vi "Multiple_File_Opener_Tester2.vi"() -> ()   [LabVIEW 2023]
uses:
  <vilib>/Utility/file.llb/Read Delimited Spreadsheet (string).vi
  <vilib>/Utility/file.llb/Read Delimited Spreadsheet (DBL).vi
panel:
  out "latest notification":string
  in  "Base Folder 2":path=path "C:/Users/AIIH/Documents/LabVIEW/EEG/Filtered_Data"
  in  "Boolean":bool
  in  "Files":path=path "C:/Users/AIIH/Documents/LabVIEW/EEG/RECORDS_1.csv"
  in  "stop":bool
  out "Header of EEGs":string[](array[string])
  out "Dataset of EEGs":dbl[][](array[numeric])
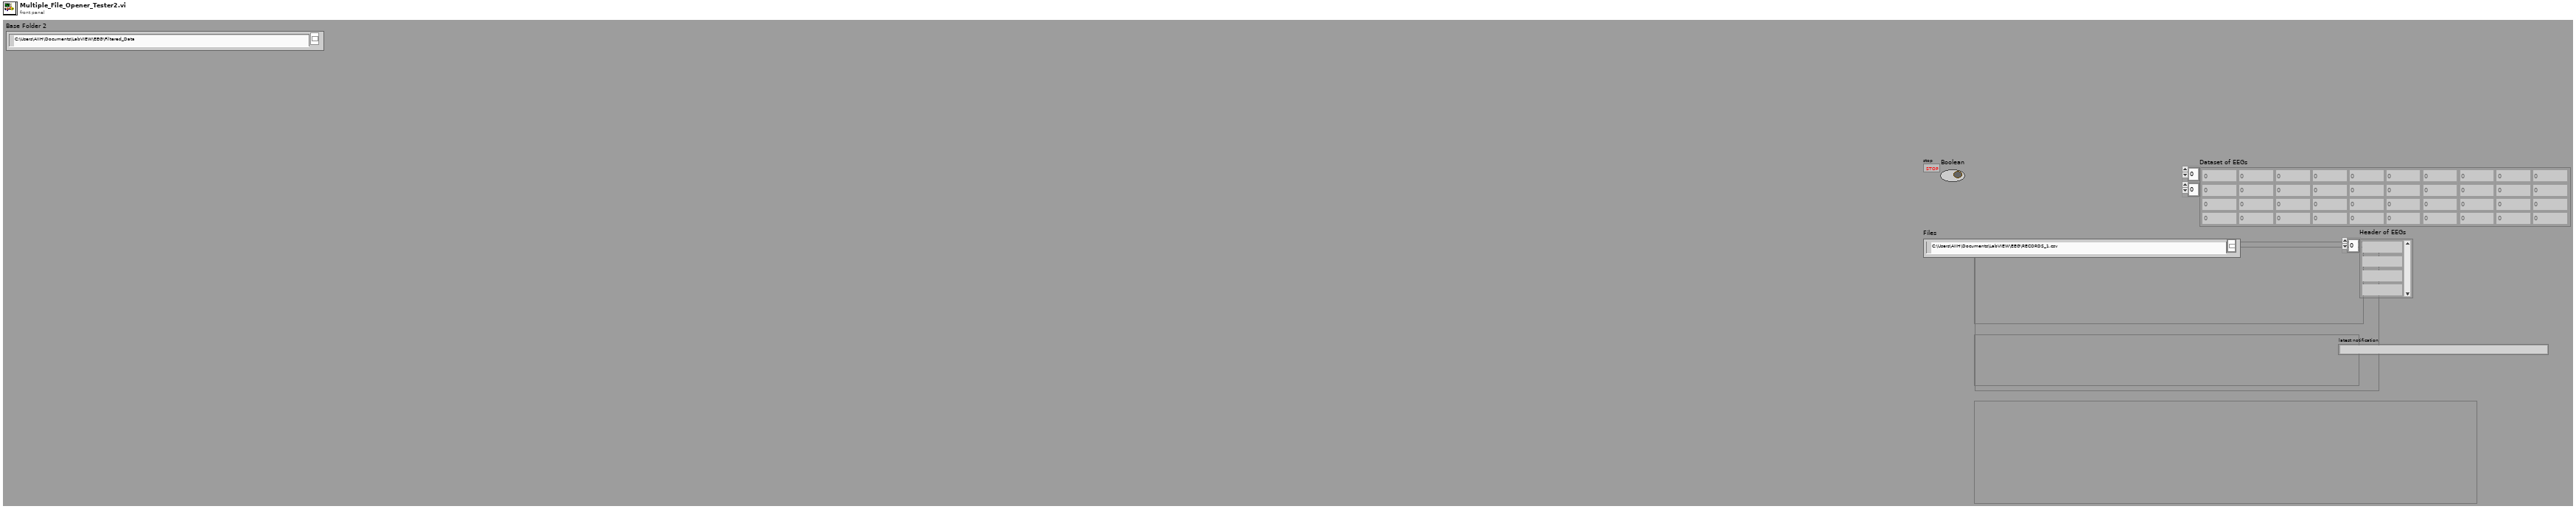
[diagram p1: front panel]
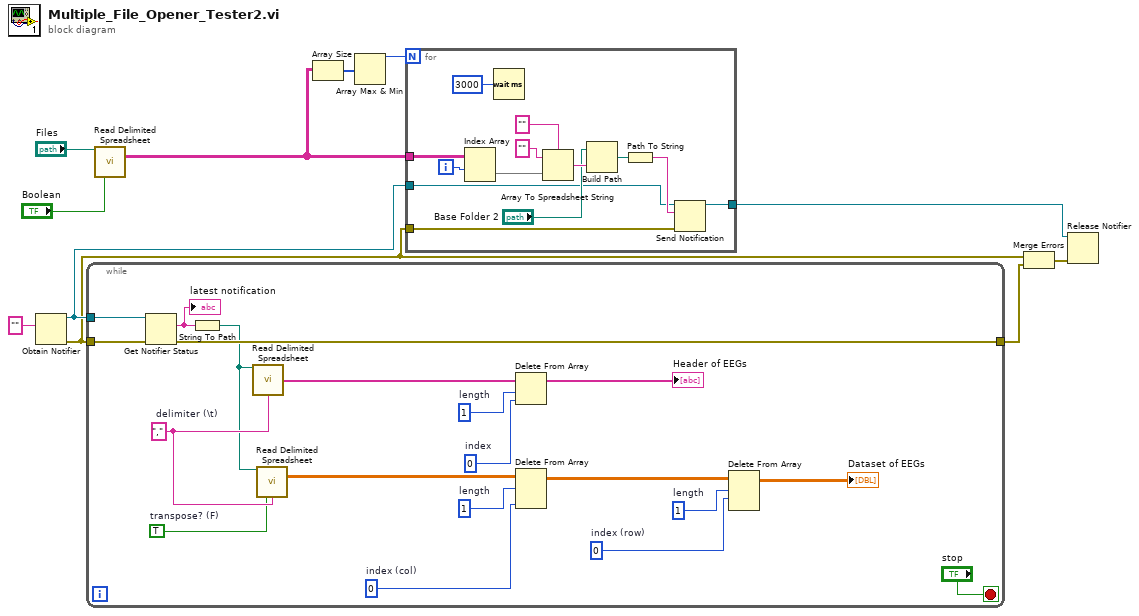
[diagram p0: block diagram]
diagram:
  n1 = Obtain Notifier(notification data type="") -> (notifier out=w4:refnum<notifier>, error out=w3:errorcluster)  [unwired: 3 in, 1 out]
  n2 = while {
    tunnel: w3 -> [w16]
    tunnel: w4 -> [w15]
    tunnel: [w14] -> w1
    stop <- "stop" stop-if-true
    w19 = TRUE  # transpose? (F)
    w20 = 0  # index
    w21 = 1  # length
    w24 = 0  # index (row)
    w25 = 1  # length
    w27 = 0  # index (col)
    w28 = 1  # length
    w30 = ","  # delimiter (\t)
    n3 = Get Notifier Status(notifier=w15, error in (no error)=w16) -> (current notification=w13:string, error out=w14:errorcluster)  [unwired: 3 out]
    "latest notification" <- w13
    n4 = String To Path(string=w13) -> (path=w12:path)
    n5 = call-poly <vilib>:"Read Delimited Spreadsheet.vi"("file path (dialog if empty)"=w12, "delimiter (\\t)"=w30) -> ("first row"=w23:string[])  [unwired: 8 in, 5 out]
    n6 = call-poly <vilib>:"Read Delimited Spreadsheet.vi"("file path (dialog if empty)"=w12, "transpose? (F)"=w19, "delimiter (\\t)"=w30) -> ("all rows"=w29:dbl[][])  [unwired: 7 in, 5 out]
    n7 = Delete From Array "Delete From Array"(array=w23, length=w21, index=w20) -> (array with subset deleted=→"Header of EEGs":string[])  [unwired: 1 out]
    n8 = Delete From Array "Delete From Array"(array=w29, length=w28, index (col)=w27) -> (array with subset deleted=w26:dbl[][])  [unwired: 1 in, 1 out]
    n9 = Delete From Array "Delete From Array"(array=w26, length=w25, index (row)=w24) -> (array with subset deleted=→"Dataset of EEGs":dbl[][])  [unwired: 1 in, 1 out]
  }
  n10 = call-poly <vilib>:"Read Delimited Spreadsheet.vi"("file path (dialog if empty)"="Files", "transpose? (F)"="Boolean") -> ("all rows"=w9:string[][])  [unwired: 8 in, 5 out]
  n11 = Array Size(array=w9) -> (size(s)=w8:i32[])
  n12 = Array Max & Min(array=w8) -> (max value=w7:i32)  [unwired: 3 out]
  n13 = for {
    N: w7 -> [_]
    tunnel: w9 -> [w43]
    tunnel: w3 -> [w33]
    tunnel: w4 -> [w32]
    tunnel: [w31] -> w5
    i -> [w42]
    n14 = Index Array(array=w43, index (row)=w42) -> (element=w39:string[])  [unwired: 1 in]
    n15 = Wait (ms)(milliseconds to wait=u32 3000) -> ()  [unwired: 1 out]
    n16 = Array To Spreadsheet String(delimiter (Tab)="", array=w39, 3:"" ("format string")) -> (spreadsheet string=w40:string)
    n17 = Build Path(base path="Base Folder 2", name or relative path=w40) -> (appended path=w35:path)
    n18 = Path To String(path=w35) -> (string=w34:string)
    n19 = Send Notification(notification=w34, notifier=w32, error in (no error)=w33) -> (notifier out=w31:refnum<notifier>)  [unwired: 1 out]
  }
  n20 = Merge Errors(w3, w1) -> (w2:errorcluster)
  n21 = Release Notifier(notifier=w5, error in (no error)=w2) -> ()  [unwired: 1 in, 3 out]
